vi "splitInput2.vi"(11 "Array":dbl[](array[numeric])) -> (2 "Defromasjon":dbl[](array[numeric]), 3 "Volt":dbl[](array[numeric]))   [LabVIEW 2015]
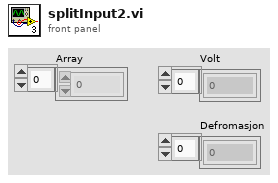
[diagram p1: front panel]
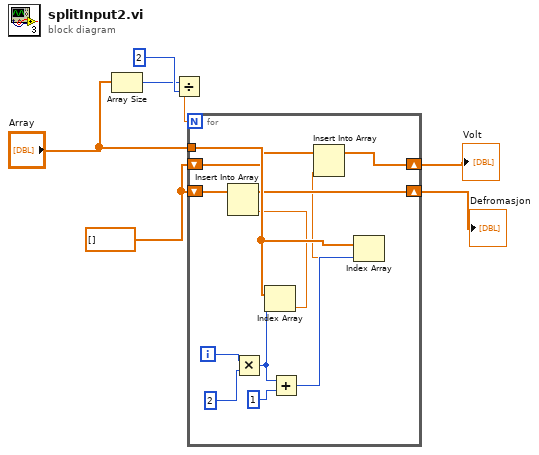
[diagram p0: block diagram]
diagram:
  w5 = dbl[] [] ("Array 2")
  n1 = Array Size(array="Array") -> (size(s)=w1:i32)
  n2 = Divide(x=w1, y=2 ("Numeric")) -> (x/y=w3:dbl)
  n3 = for {
    N: w3 -> [_]
    tunnel: "Array" -> [w14]
    shift-right: [w11] -> w7
    shift-left: w5 -> [w13]
    shift-right: [w8] -> w6
    shift-left: w5 -> [w10]
    i -> [w16]
    n4 = Multiply(x=w16, y=2 ("Numeric")) -> (x*y=w18:i32)
    n5 = Index Array(array=w14, index=w18) -> (element=w12:dbl)
    n6 = Insert Into Array(array=w13, new element=w12) -> (w11:dbl[])  [unwired: 1 in]
    n7 = Add(x=w18, y=1) -> (x+y=w15:i32)
    n8 = Index Array(array=w14, index=w15) -> (element=w9:dbl)
    n9 = Insert Into Array(array=w10, new element=w9) -> (w8:dbl[])  [unwired: 1 in]
  }
  "Volt" <- w6
  "Defromasjon" <- w7
